vi "Generate SQL Query.vi"(4 "Order by":T1, 5 "Extra cmd":string, 6 "Query type":T2, 7 "Where Statement":cluster{"Value":string, "Condition":string}[](array[cluster]), 8 "error in (no error)":errorcluster, 9 "Values":string[](array[string]), 10 "Column Name":string[](array[string]), 11 "Table Name":string) -> (0 "error out":errorcluster, 2 "Query String":string="SELECT `config_name`,`value` FROM `configuration` ORDER BY `id` ASC ")   [LabVIEW 2020]
uses:
  Control/State - Query Type.ctl
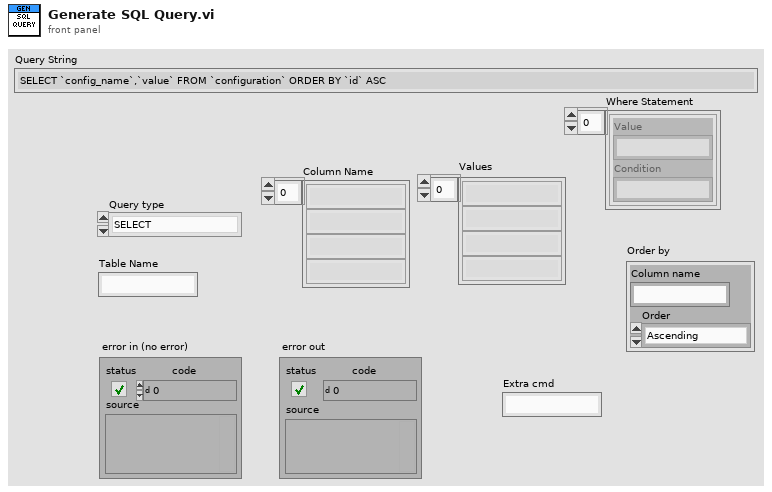
[diagram p1: front panel]
types:
  T1 = cluster{"Column name":string, "Order":enum16{"Ascending", "Descending"}}
  T2 = typedef "State - Query Type.ctl" = enum16{"SELECT", "UPDATE", "INSERT INTO", "TRUNCATE TABLE"}
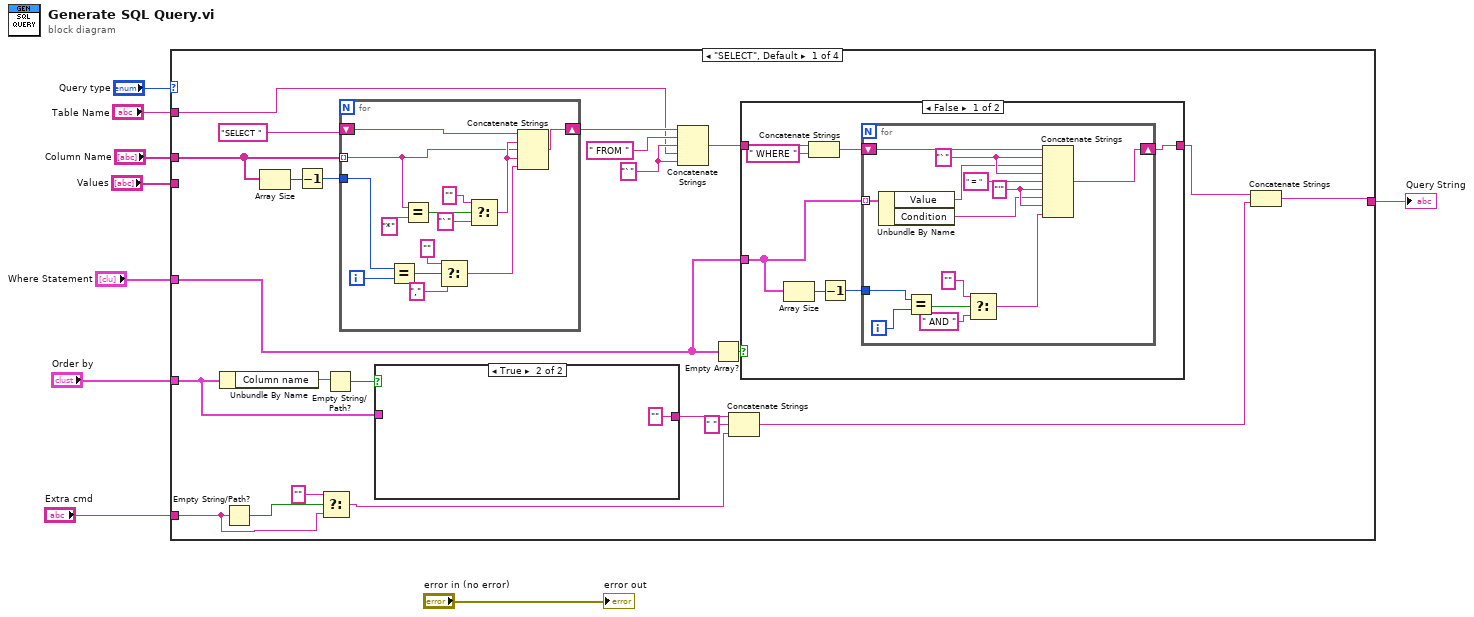
[diagram p0: block diagram]
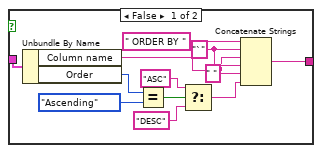
[diagram p2: hidden frame]
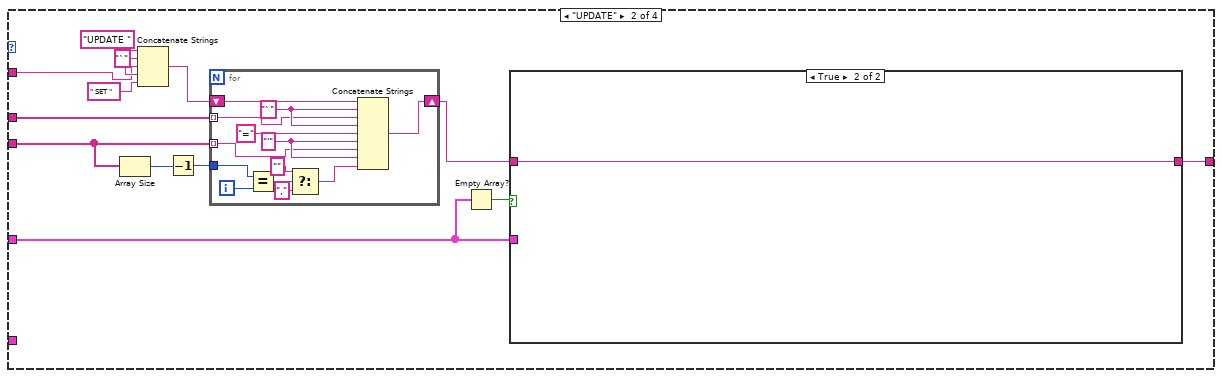
[diagram p4: hidden frame]
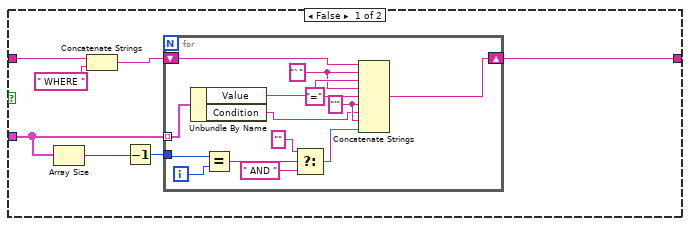
[diagram p5: hidden frame]
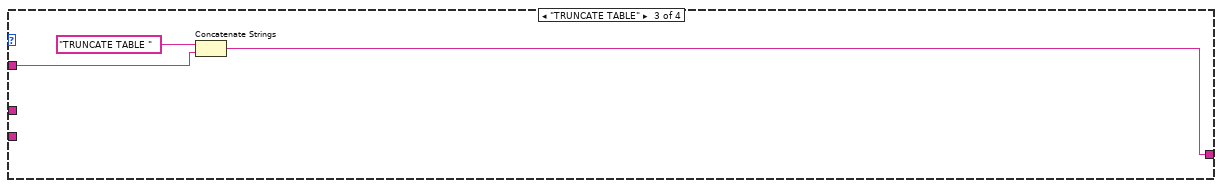
[diagram p6: hidden frame]
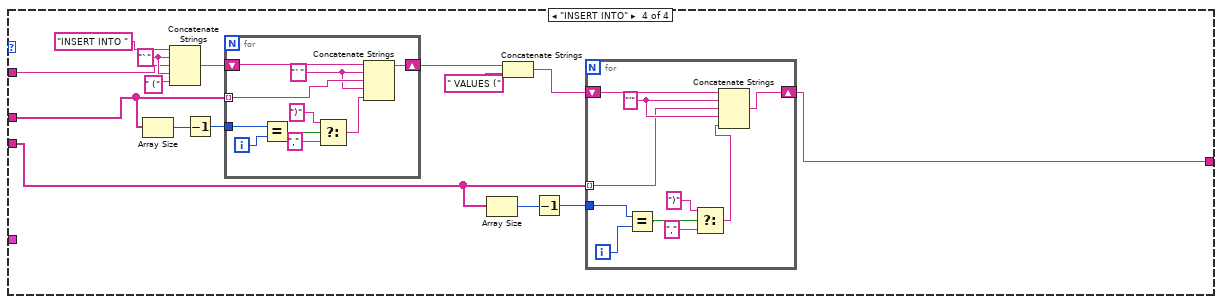
[diagram p7: hidden frame]
diagram:
  n1 = case shown="\"SELECT\", Default" "Query type" {
    tunnel: "Table Name" -> [w25 w85 w131 w145]
    tunnel: "Column Name" -> [w32 w93 _ w142]
    tunnel: "Values" -> [_ w91 _ w137]
    tunnel: "Where Statement" -> [w22 w82 _ _]
    tunnel: [w20 w87 w130 w133] -> w3
    tunnel: "Order by" -> [w17 _ _ _]
    tunnel: "Extra cmd" -> [w12 _ _ _]
    frame "SELECT", Default {
      w26 = "`" ("string")
      n2 = Unbundle By Name(w17) -> ("Column name"=w19:string)
      n3 = Empty String/Path?(string/path=w12) -> (empty?=w13:bool)
      n4 = Array Size(array=w32) -> (size(s)=w31:i32)
      n5 = Decrement(x=w31) -> (x-1=w30:i32)
      n6 = Select(t="", s=w13, f=w12) -> (s? t:f=w10:string)
      n7 = Empty String/Path?(string/path=w19) -> (empty?=w18:bool)
      n8 = for {
        tunnel: w32 -> [w69] mode=indexing
        shift-right: [w72] -> w29
        shift-left: "SELECT " ("string") -> [w71]
        tunnel: w30 -> [w81]
        i -> [w80]
        n9 = Equal?(x=w81, y=w80) -> (x = y?=w78:bool)
        n10 = Equal?(x=w69, y="*") -> (x = y?=w75:bool)
        n11 = Select(t="", s=w78, f=",") -> (s? t:f=w68:string)
        n12 = Select(t="", s=w75, f="`") -> (s? t:f=w70:string)
        n13 = Concatenate Strings(w71, w70, w69, w70, w68) -> (w72:string)
      }
      n14 = case shown="True" w18 {
        tunnel: w17 -> [w44 _]
        tunnel: [w33 ""] -> w16
        frame False {
          w42 = "`" ("string")
          n15 = Unbundle By Name(w44) -> ("Column name"=w41:string, "Order"=w39:enum16{"Ascending", "Descending"})
          n16 = Equal?(x=w39, y=enum16{"Ascending", "Descending"}."Ascending") -> (x = y?=w37:bool)
          n17 = Select(t="ASC" ("string"), s=w37, f="DESC") -> (s? t:f=w34:string)
          n18 = Concatenate Strings(" ORDER BY " ("string"), w42, w41, w42, " " ("string"), w34) -> (w33:string)
        }
        frame True {
        }
      }
      n19 = Concatenate Strings(w29, " FROM " ("string"), w26, w25, w26) -> (w24:string)
      n20 = Empty Array?(array=w22) -> (empty?=w23:bool)
      n21 = Concatenate Strings(w16, " " ("string"), w10) -> (w14:string)
      n22 = case shown="False" w23 {
        tunnel: w24 -> [w52 w67]
        tunnel: [w46 w67] -> w21
        tunnel: w22 -> [w49 _]
        frame False {
          n23 = Array Size(array=w49) -> (size(s)=w48:i32)
          n24 = Concatenate Strings(w52, " WHERE " ("string")) -> (w50:string)
          n25 = Decrement(x=w48) -> (x-1=w47:i32)
          n26 = for {
            tunnel: w49 -> [w66] mode=indexing
            shift-right: [w57] -> w46
            shift-left: w50 -> [w65]
            tunnel: w47 -> [w63]
            i -> [w64]
            w59 = "'" ("string")
            w62 = "`" ("string")
            n27 = Unbundle By Name(w66) -> ("Value"=w61:string, "Condition"=w58:string)
            n28 = Equal?(x=w63, y=w64) -> (x = y?=w56:bool)
            n29 = Select(t="" ("string"), s=w56, f=" AND ") -> (s? t:f=w53:string)
            n30 = Concatenate Strings(w65, w62, w61, w62, " = " ("string"), w59, w58, w59, w53) -> (w57:string)
          }
        }
        frame True {
        }
      }
      n31 = Concatenate Strings(w21, w14) -> (w20:string)
    }
    frame "UPDATE" {
      w86 = "`" ("string")
      n32 = Array Size(array=w91) -> (size(s)=w90:i32)
      n33 = Concatenate Strings("UPDATE ", w86, w85, w86, " SET ") -> (w92:string)
      n34 = Decrement(x=w90) -> (x-1=w89:i32)
      n35 = for {
        tunnel: w93 -> [w126] mode=indexing
        tunnel: w91 -> [w123] mode=indexing
        shift-right: [w128] -> w88
        shift-left: w92 -> [w129]
        tunnel: w89 -> [w121]
        i -> [w122]
        w124 = "'" ("string")
        w127 = "`" ("string")
        n36 = Equal?(x=w121, y=w122) -> (x = y?=w120:bool)
        n37 = Select(t="" ("string"), s=w120, f=",") -> (s? t:f=w117:string)
        n38 = Concatenate Strings(w129, w127, w126, w127, "=" ("string"), w124, w123, w124, w117) -> (w128:string)
      }
      n39 = Empty Array?(array=w82) -> (empty?=w83:bool)
      n40 = case shown="True" w83 {
        tunnel: w88 -> [w101 w116]
        tunnel: w82 -> [w99 _]
        tunnel: [w96 w116] -> w87
        frame False {
          n41 = Array Size(array=w99) -> (size(s)=w98:i32)
          n42 = Concatenate Strings(w101, " WHERE " ("string")) -> (w100:string)
          n43 = Decrement(x=w98) -> (x-1=w97:i32)
          n44 = for {
            tunnel: w99 -> [w115] mode=indexing
            shift-right: [w102] -> w96
            shift-left: w100 -> [w114]
            tunnel: w97 -> [w108]
            i -> [w107]
            w110 = "'" ("string")
            w112 = "`" ("string")
            n45 = Unbundle By Name(w115) -> ("Value"=w113:string, "Condition"=w109:string)
            n46 = Equal?(x=w108, y=w107) -> (x = y?=w106:bool)
            n47 = Select(t="" ("string"), s=w106, f=" AND ") -> (s? t:f=w103:string)
            n48 = Concatenate Strings(w114, w112, w113, w112, "=" ("string"), w110, w109, w110, w103) -> (w102:string)
          }
        }
        frame True {
        }
      }
    }
    frame "TRUNCATE TABLE" {
      n49 = Concatenate Strings("TRUNCATE TABLE " ("string"), w131) -> (w130:string)
    }
    frame "INSERT INTO" {
      w146 = "`" ("string")
      n50 = Array Size(array=w142) -> (size(s)=w141:i32)
      n51 = Concatenate Strings("INSERT INTO " ("string"), w146, w145, w146, " (" ("string")) -> (w143:string)
      n52 = Decrement(x=w141) -> (x-1=w140:i32)
      n53 = for {
        tunnel: w142 -> [w161] mode=indexing
        shift-right: [w159] -> w139
        shift-left: w143 -> [w162]
        tunnel: w140 -> [w166]
        i -> [w167]
        w160 = "`" ("string")
        n54 = Equal?(x=w166, y=w167) -> (x = y?=w165:bool)
        n55 = Select(t=")", s=w165, f=",") -> (s? t:f=w158:string)
        n56 = Concatenate Strings(w162, w160, w161, w160, w158) -> (w159:string)
      }
      n57 = Array Size(array=w137) -> (size(s)=w136:i32)
      n58 = Concatenate Strings(w139, " VALUES (" ("string")) -> (w134:string)
      n59 = Decrement(x=w136) -> (x-1=w135:i32)
      n60 = for {
        tunnel: w137 -> [w150] mode=indexing
        tunnel: w135 -> [w157]
        shift-right: [w148] -> w133
        shift-left: w134 -> [w152]
        i -> [w156]
        w151 = "'" ("string")
        n61 = Equal?(x=w157, y=w156) -> (x = y?=w154:bool)
        n62 = Select(t=")", s=w154, f=",") -> (s? t:f=w149:string)
        n63 = Concatenate Strings(w152, w151, w150, w151, w149) -> (w148:string)
      }
    }
  }
  "Query String" <- w3
  "error out" <- "error in (no error)"
